vi "Temp Server.vi"() -> ()   [LabVIEW 2024]
panel:
  in  "Max. Temp Set Point":i32(knob)=70 scale=60.0..80.0
  in  "Lower. Temp Set Point":i32(knob)=40 scale=40.0..60.0
  out "Waveform Chart":dynamicdata(graph)
  out "Thermometer":dbl(slide) scale=0.0..100.0
  out "Heater":bool
  in  "Iteration Rate":u32=200
  in  "stop":bool
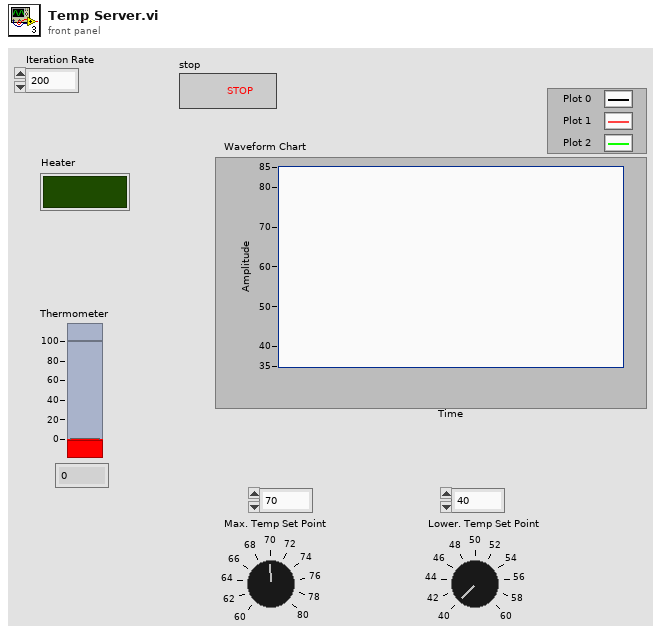
[diagram p1: front panel]
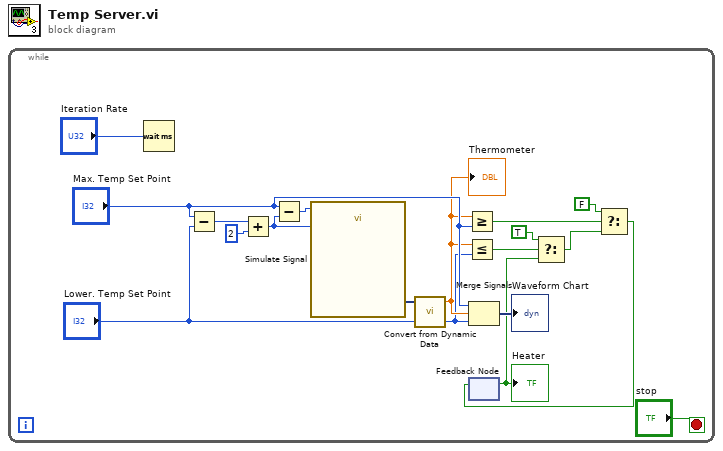
[diagram p0: block diagram]
diagram:
  n1 = while {
    stop <- "stop" stop-if-true
    n2 = Wait (ms)(milliseconds to wait="Iteration Rate") -> ()  [unwired: 1 out]
    n3 = Subtract(x="Max. Temp Set Point", y="Lower. Temp Set Point") -> (x-y=w18:i32)
    n4 = Add(x=w18, y=2) -> (x+y=w16:i32)
    n5 = Subtract(x="Max. Temp Set Point", y=w16) -> (x-y=w15:i32)
    n6 = call "Simulate Signal"("Offset"=w15, "Amplitude"=w16) -> ("Sine with Uniform Noise"=w14:dynamicdata)  [unwired: 12 in, 1 out]
    n7 = call "Convert from Dynamic Data"("Dynamic Data Type"=w14) -> ("Scalar"=w11:dbl)  [unwired: 3 in]
    "Thermometer" <- w11
    n8 = Greater Or Equal?(x=w11, y="Max. Temp Set Point") -> (x >= y?=w9:bool)
    n9 = Less Or Equal?(x=w11, y="Lower. Temp Set Point") -> (x <= y?=w8:bool)
    n10 = Merge Signals("Max. Temp Set Point", w11, "Lower. Temp Set Point") -> (→"Waveform Chart":dynamicdata)
    n11 = feedback #1() -> (w3:bool)  [unwired: 1 in]
    "Heater" <- w3
    n12 = Select(t=TRUE, s=w8, f=w3) -> (s? t:f=w5:bool)
    n13 = Select(t=FALSE, s=w9, f=w5) -> (s? t:f=w4:bool)
    n14 = feedback-in #1(w4) -> ()
  }
